vi "MFC Settings (SubVI).vi"(0 "N2 Control":refnum<vi>, 1 "NOx Control":refnum<vi>, 2 "Channel Names":string[](array[string]), 3 "VOC Control":refnum<vi>, 4 "N2 Display":refnum<vi>, 5 "error in (no error)":errorcluster, 6 "O2 Control":refnum<vi>, 7 "O2 Display":refnum<vi>, 8 "# RH Probes":i32, 9 "VOC Display":refnum<vi>, 10 "# RH (T) Probes":i32, 11 "NOx Display":refnum<vi>, 12 "# Channels":i32, 13 "task in":refnum<k21>) -> (14 "Refnum out":refnum<k21>, 16 "MFC Units":string[](array[string]), 19 "error out":errorcluster)   [LabVIEW 2011]
uses:
  <vilib>/Utility/error.llb/DialogType.ctl
  Program Files (x86)/National Instruments/LabVIEW 2011/resource/objmgr/daqmx.rc
panel:
  in  "Array - String":string[](array[string])
  out "Min Scale Values":dbl[](array[numeric])
  out "Max Scale Values":dbl[](array[numeric])
  # "INPUTS"
  # "All Incoming Channel Names from NI Board"
  # "OUTPUTS"
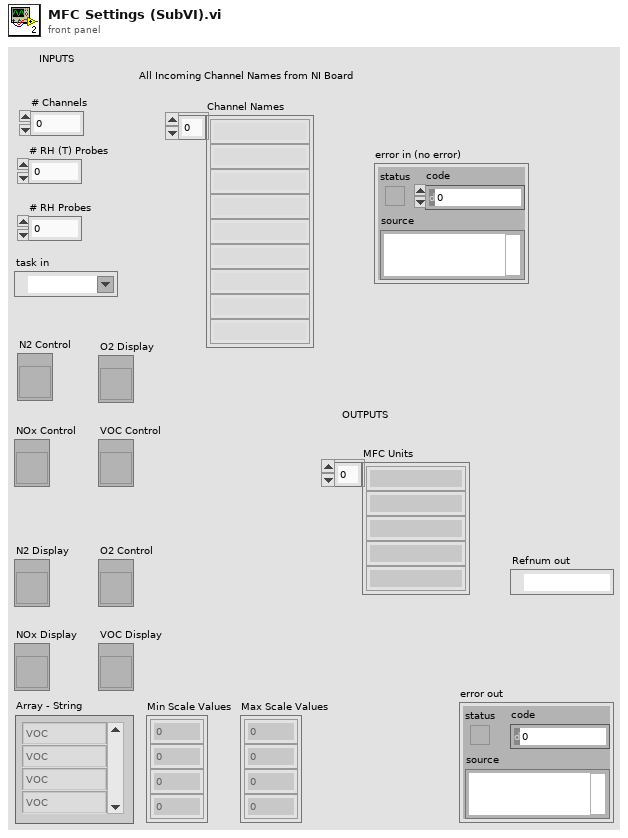
[diagram p1: front panel]
types:
  T1 = typedef "DialogType.ctl" = u16
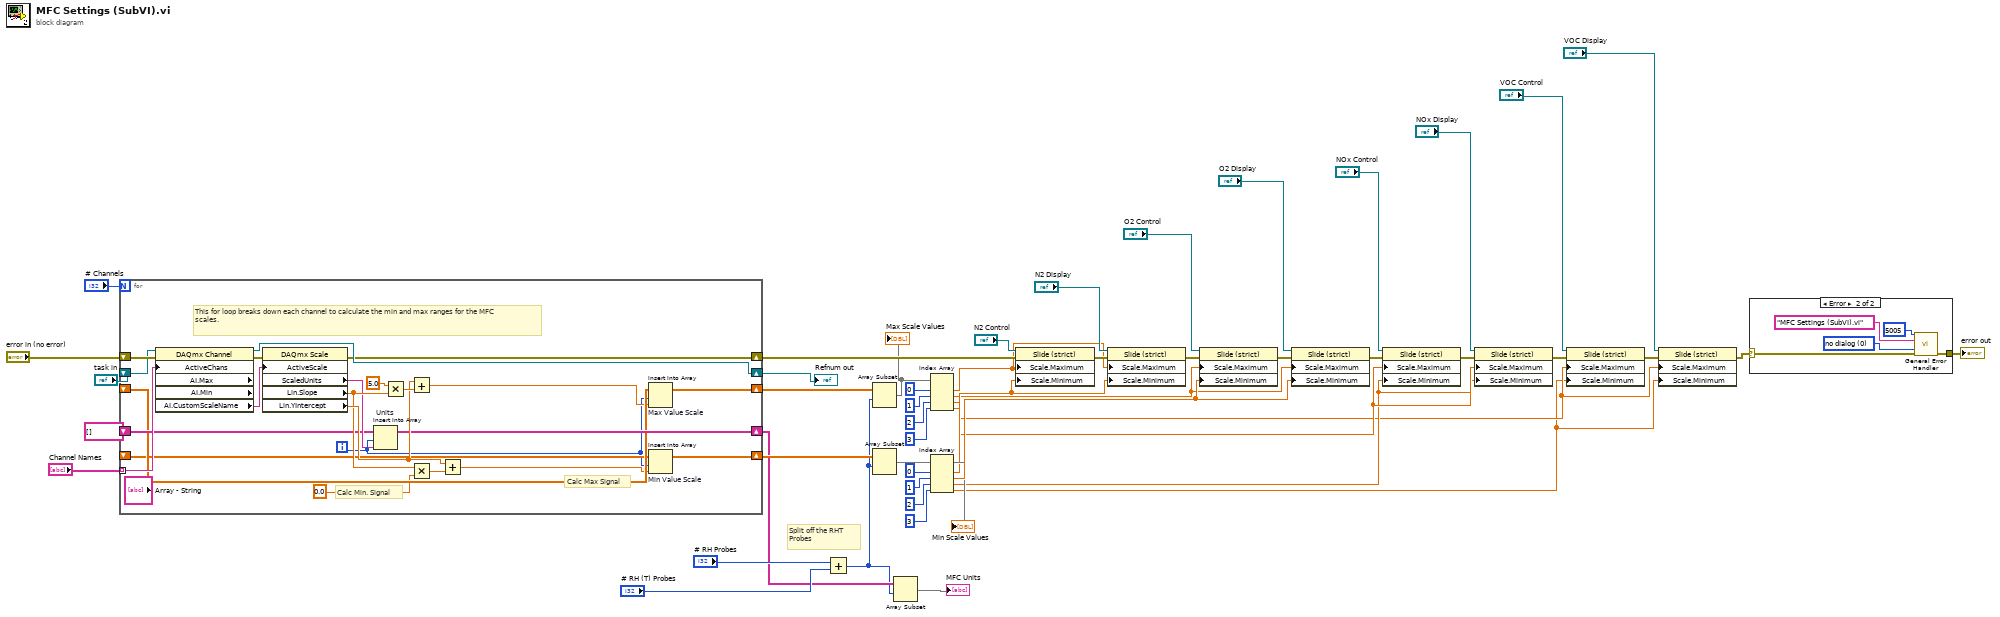
[diagram p0: block diagram]
diagram:
  # "Split off the RHT Probes"
  n1 = for {
    N: "# Channels" -> [_]
    shift-right: [w50] -> w49
    shift-left: "error in (no error)" -> [w71]
    shift-right: [w69] -> w24
    shift-left: "task in" -> [w68]
    tunnel: "Channel Names" -> [w63] mode=indexing
    shift-right: [w62] -> w26
    shift-left: _ -> [w58]
    shift-right: [w60] -> w15
    shift-left: string[] [] -> [w59]
    shift-right: [w56] -> w39
    shift-left: _ -> [w55]
    i -> [w53]
    # "This for loop breaks down each channel to calculate the min and max ranges for the MFC scales."
    # "Calc Min. Signal"
    # "Calc Max Signal"
    n2 = property class="DAQmx Channel" props=["ActiveChans", "AI.Max", "AI.Min", "AI.CustomScaleName"](reference=w68, error in=w71, "ActiveChans"=w63) -> (reference out=w69:refnum<k21>, error out=w72:errorcluster, "AI.CustomScaleName"=w70:tag)  [unwired: 2 out]
    n3 = property class="DAQmx Scale"(error in=w72, "ActiveScale"=w70) -> (error out=w50:errorcluster, "ScaledUnits"=w61:string, "Lin.Slope"=w64:dbl, "Lin.YIntercept"=w65:dbl)  [unwired: 1 in, 1 out]
    n4 = Insert Into Array "Units"(array=w59, index=w53, new element=w61) -> (w60:string[])
    n5 = Multiply(x=5.0 ("new element/subarray"), y=w64) -> (x*y=w67:dbl)
    n6 = Add(x=w65, y=w67) -> (x+y=w57:dbl)
    n7 = Multiply(x=w64, y=0.0 ("new element/subarray")) -> (x*y=w66:dbl)
    n8 = Add(x=w65, y=w66) -> (x+y=w54:dbl)
    n9 = Insert Into Array "Max Value Scale"(array=w58, index=w53, new element=w57) -> (w62:dbl[])
    n10 = Insert Into Array "Min Value Scale"(array=w55, index=w53, new element=w54) -> (w56:dbl[])
  }
  "Refnum out" <- w24
  n11 = Add(x="# RH Probes", y="# RH (T) Probes") -> (x+y=w14:i32)
  n12 = Array Subset(array=w26, index=w14) -> (w27:dbl[])  [unwired: 1 in]
  "Max Scale Values" <- w27
  n13 = Array Subset(array=w39, index=w14) -> (w40:dbl[])  [unwired: 1 in]
  "Min Scale Values" <- w40
  n14 = Array Subset(array=w15, index=w14) -> (→"MFC Units":string[])  [unwired: 1 in]
  n15 = Index Array(array=w27, index #1=0 ("index"), index #2=1 ("index"), index #3=2 ("index"), index #4=3 ("index")) -> (element #1=w10:dbl, element #2=w9:dbl, element #3=w8:dbl, element #4=w6:dbl)
  n16 = Index Array(array=w40, index #1=0 ("index"), index #2=1 ("index"), index #3=2 ("index"), index #4=3 ("index")) -> (element #1=w11:dbl, element #2=w41:dbl, element #3=w7:dbl, element #4=w5:dbl)
  n17 = property on="Property Node" class="Slide (strict)"(reference="N2 Control", error in=w49, "Scale.Maximum"=w10, "Scale.Minimum"=w11) -> (error out=w42:errorcluster)  [unwired: 1 out]
  n18 = property on="Property Node" class="Slide (strict)"(reference="N2 Display", error in=w42, "Scale.Maximum"=w10, "Scale.Minimum"=w11) -> (error out=w43:errorcluster)  [unwired: 1 out]
  n19 = property on="Property Node" class="Slide (strict)"(reference="O2 Control", error in=w43, "Scale.Maximum"=w9, "Scale.Minimum"=w41) -> (error out=w44:errorcluster)  [unwired: 1 out]
  n20 = property on="Property Node" class="Slide (strict)"(reference="O2 Display", error in=w44, "Scale.Maximum"=w9, "Scale.Minimum"=w41) -> (error out=w45:errorcluster)  [unwired: 1 out]
  n21 = property on="Property Node" class="Slide (strict)"(reference="NOx Control", error in=w45, "Scale.Maximum"=w8, "Scale.Minimum"=w7) -> (error out=w46:errorcluster)  [unwired: 1 out]
  n22 = property on="Property Node" class="Slide (strict)"(reference="NOx Display", error in=w46, "Scale.Maximum"=w8, "Scale.Minimum"=w7) -> (error out=w47:errorcluster)  [unwired: 1 out]
  n23 = property on="Property Node" class="Slide (strict)"(reference="VOC Control", error in=w47, "Scale.Maximum"=w6, "Scale.Minimum"=w5) -> (error out=w48:errorcluster)  [unwired: 1 out]
  n24 = property on="Property Node" class="Slide (strict)"(reference="VOC Display", error in=w48, "Scale.Maximum"=w6, "Scale.Minimum"=w5) -> (error out=w17:errorcluster)  [unwired: 1 out]
  n25 = case shown="Error" w17 {
    selector: w17 -> [w73 w78]
    tunnel: [w73 w77] -> w16
    frame No Error {
    }
    frame Error {
      w74 = T1 0 items=["no dialog", "OK message", "continue or stop message", "OK message + warnings", "continue/stop + warnings"] ("type of dialog (OK msg:1)")
      n26 = call <vilib>:"General Error Handler.vi"("[error code] (0)"=5005, "[error source] (\" \")"="MFC Settings (SubVI).vi" ("[error source] (\" \")"), "type of dialog (OK msg:1)"=w74, "error in (no error)"=w78) -> ("error out"=w77:errorcluster)  [unwired: 7 in, 4 out]
    }
  }
  "error out" <- w16
